vi "Load Becker-Hickl Data.vi"(8 "Error In":errorcluster, 9 "Data Block Types":T2[](array[typedef]), 10 "Data Block Headers":T5[](array[typedef]) {"Block Type" format="%.0b"; "Long Block Number" format="%.0b"}, 11 "File Path Control":path) -> (0 "Error Out":errorcluster, 2 "Block Contents":T1[](array[typedef]), 3 "Data Blocks":sgl[][](array[numeric]))   [LabVIEW 2021, in "Becker-Hickl Files.lvlib"]
uses:
  Becker-Hickl Files.lvlib
  Becker-Hickl Data Block Header.ctl
  Becker-Hickl Data Creation Mode.ctl
  Becker-Hickl Data Block Content.ctl
  Becker-Hickl Data Type.ctl
  Becker-Hickl Data Block Type.ctl
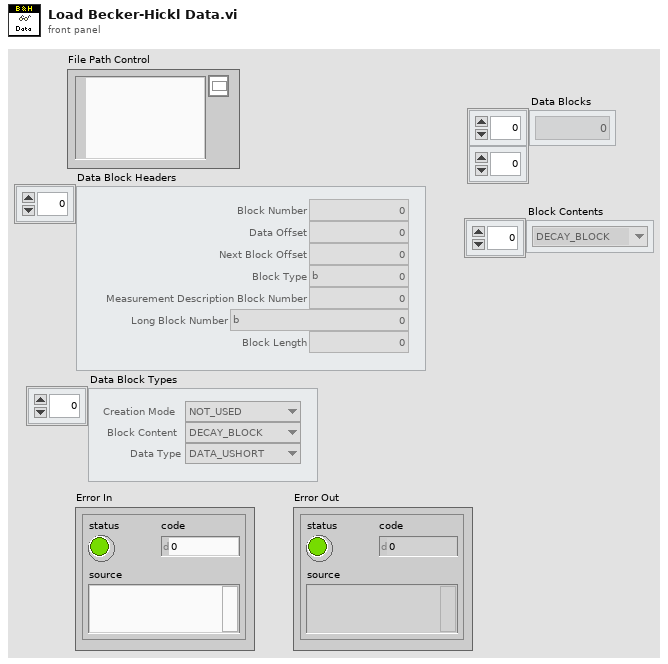
[diagram p1: front panel]
types:
  T1 = typedef "Becker-Hickl Files.lvlib/Becker-Hickl Data Block Content.ctl" = enum16{"DECAY_BLOCK", "PAGE_BLOCK", "FCS_BLOCK", "FIDA_BLOCK", "FILDA_BLOCK", "MCS_BLOCK", "IMG_BLOCK"}
  T2 = typedef "Becker-Hickl Files.lvlib/Becker-Hickl Data Block Type.ctl" = cluster{"Creation Mode":T3, "Block Content":T1, "Data Type":T4}
  T3 = typedef "Becker-Hickl Files.lvlib/Becker-Hickl Data Creation Mode.ctl" = enum16{"NOT_USED", "MEAS_DATA", "FLOW_DATA", "MEAS_DATA_FROM_FILE", "CALC_DATA", "SIM_DATA", "FIFO_DATA", "FIFO_DATA_FROM_FILE"}
  T4 = typedef "Becker-Hickl Files.lvlib/Becker-Hickl Data Type.ctl" = enum16{"DATA_USHORT", "DATA_ULONG", "DATA_DBL"}
  T5 = typedef "Becker-Hickl Files.lvlib/Becker-Hickl Data Block Header.ctl" = cluster{"Block Number":u16, "Data Offset":u32, "Next Block Offset":u32, "Block Type":u16, "Measurement Description Block Number":u16, "Long Block Number":u32, "Block Length":u32}
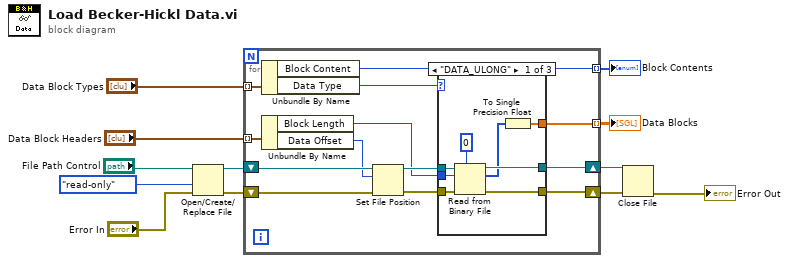
[diagram p0: block diagram]
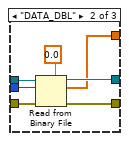
[diagram p2: hidden frame]
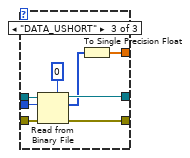
[diagram p3: hidden frame]
diagram:
  n1 = Open/Create/Replace File(file path (use dialog)="File Path Control", error in="Error In", access (0:read/write)=enum16{"read/write", "read-only", "write-only"}."read-only") -> (refnum out=w8:refnum<file>, error out=w7:errorcluster)  [unwired: 3 in, 1 out]
  n2 = for {
    tunnel: "Data Block Headers" -> [w25] mode=indexing
    shift-right: [w23] -> w4
    shift-left: w7 -> [w21]
    tunnel: "Data Block Types" -> [w17] mode=indexing
    shift-right: [w15] -> w5
    shift-left: w8 -> [w24]
    tunnel: [w14] -> w1 mode=indexing
    tunnel: [w13] -> w2 mode=indexing
    n3 = Unbundle By Name(w17) -> ("Block Content"=w13:T1, "Data Type"=w16:T4)
    n4 = Unbundle By Name(w25) -> ("Block Length"=w18:u32, "Data Offset"=w19:u32)
    n5 = Set File Position(offset (in bytes) (0)=w19, refnum=w24, error in=w21) -> (refnum out=w22:refnum<file>, error out=w20:errorcluster)  [unwired: 1 in]
    n6 = case shown="\"DATA_ULONG\"" w16 {
      tunnel: [w33 w40 w48] -> w23
      tunnel: w22 -> [w32 w39 w47]
      tunnel: w20 -> [w31 w38 w46]
      tunnel: w18 -> [w30 w37 w45]
      tunnel: [w28 w35 w43] -> w15
      tunnel: [w26 w34 w41] -> w14
      frame "DATA_ULONG" {
        n7 = Read from Binary File(5:u32 0, 8:w31, 10:w30, 11:w32) -> (0:w33:errorcluster, 2:w27:u32[], 3:w28:refnum<file>)  [unwired: 2 in, 1 out]
        n8 = To Single Precision Float(number=w27) -> (single precision float=w26:sgl[])
      }
      frame "DATA_DBL" {
        n9 = Read from Binary File(5:sgl 0.0, 8:w38, 10:w37, 11:w39) -> (0:w40:errorcluster, 2:w34:sgl[], 3:w35:refnum<file>)  [unwired: 2 in, 1 out]
      }
      frame "DATA_USHORT" {
        n10 = Read from Binary File(5:u16 0, 8:w46, 10:w45, 11:w47) -> (0:w48:errorcluster, 2:w42:u16[], 3:w43:refnum<file>)  [unwired: 2 in, 1 out]
        n11 = To Single Precision Float(number=w42) -> (single precision float=w41:sgl[])
      }
    }
  }
  "Block Contents" <- w2
  "Data Blocks" <- w1
  n12 = Close File(refnum=w5, error in=w4) -> (error out=→"Error Out":errorcluster)  [unwired: 1 out]
